vi "Write State.vi"(8 "error in":errorcluster, 10 "State":bool, 11 "DAQmxSwitch in":refnum<class "DAQmxSwitch.lvclass">) -> (0 "error out":errorcluster, 3 "DAQmxSwitch out":refnum<class "DAQmxSwitch.lvclass">)   [LabVIEW 2014, in "DAQmxSwitch.lvclass"]
uses:
  DAQmxSwitch.lvclass
  Switch.lvclass
  <resource>/objmgr/daqmx.rc
  <vilib>/DAQmx/read.llb/DAQmx Read (Digital 1D Bool NChan 1Samp 1Line).vi
  <vilib>/DAQmx/write.llb/DAQmx Write (Digital 1D Bool NChan 1Samp 1Line).vi
  <vilib>/DAQmx/write.llb/DAQmx Write (Digital Bool 1Line 1Point).vi
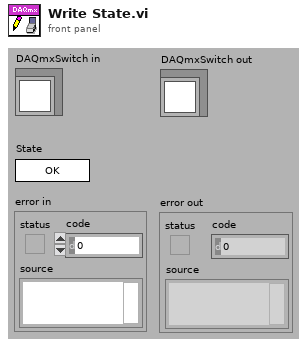
[diagram p1: front panel]
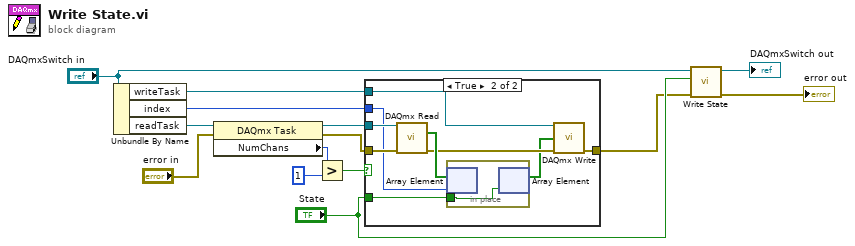
[diagram p0: block diagram]
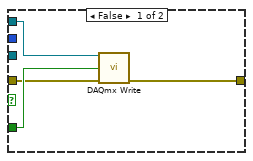
[diagram p2: hidden frame]
diagram:
  n1 = Unbundle By Name("DAQmxSwitch in") -> ("writeTask"=w1:refnum<k21>, "index"=w2:i32, "readTask"=w12:refnum<k21>)
  n2 = property class="DAQmx Task"(reference=w12, error in="error in") -> (reference out=w10:refnum<k21>, error out=w8:errorcluster, "NumChans"=w11:u32)
  n3 = Greater?(x=w11, y=u32 1) -> (0:w6:bool)
  n4 = case shown="True" w6 {
    tunnel: w10 -> [_ w27]
    tunnel: w8 -> [w17 w24]
    tunnel: "State" -> [w18 w23]
    tunnel: w2 -> [_ w21]
    tunnel: [w16 w20] -> w3
    tunnel: w1 -> [w15 w19]
    frame False {
      n5 = call-poly <vilib>:"DAQmx Write.vi"("task/channels in"=w15, "data"=w18, "error in"=w17) -> ("error out"=w16:errorcluster)  [unwired: 10 in, 2 out]
    }
    frame True {
      n6 = call-poly <vilib>:"DAQmx Read.vi"("task/channels in"=w27, "error in"=w24) -> ("data"=w26:bool[], "error out"=w25:errorcluster)  [unwired: 11 in, 1 out]
      n7 = in-place {
        in-place-border: w23 -> [w28]
        n8 = in-place-array #1(w26, w21) -> ()  [unwired: 1 out]
        n9 = in-place-array #1(w28) -> (w22:bool[])  [unwired: 1 out]
      }
      n10 = call-poly <vilib>:"DAQmx Write.vi"("task/channels in"=w19, "data"=w22, "error in"=w25) -> ("error out"=w20:errorcluster)  [unwired: 10 in, 2 out]
    }
  }
  n11 = call-parent "Write State.vi"("error in"=w3, "State"="State", "Switch in"="DAQmxSwitch in") -> ("error out"=→"error out":errorcluster, "Switch out"=→"DAQmxSwitch out":refnum<class "DAQmxSwitch.lvclass">)  [unwired: 7 in]
